vi "sv_UFF58 Create Function and Channels.vi"(0 "file refnum":refnum<k20>, 1 "real or complex data?":enum16{"Real data", "Complex data"}(ring), 11 "error in (no error)":errorcluster) -> (4 "dup file refnum":refnum<k20>, 6 "function refnum":refnum<k20>, 8 "channel refnums":refnum<k20>[](array[refnum]), 12 "ordinate denominator channel name":string, 13 "ordinate numerator channel name":string, 14 "abscissa channel name":string, 15 "error out":errorcluster)   [LabVIEW 2017, in "SoundVib_UFF58.lvlib"]
doc: "This VI creates a new <B>function refnum</B>. It also creates multiple <B>channel refnums</B> depending on the value of <B>real or complex data?</B>. If real, only two channels are created (X and Y). If complex, three channels are created (X, Yreal, and Yimag)."
uses:
  <vilib>/addons/Sound and Vibration/svt_UFF58/SoundVib_UFF58.lvlib
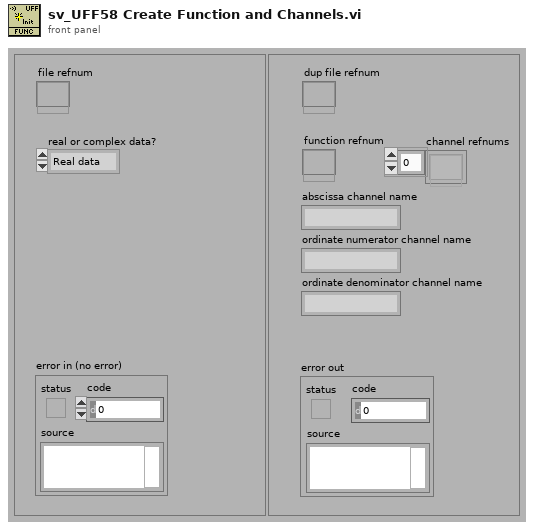
[diagram p1: front panel]
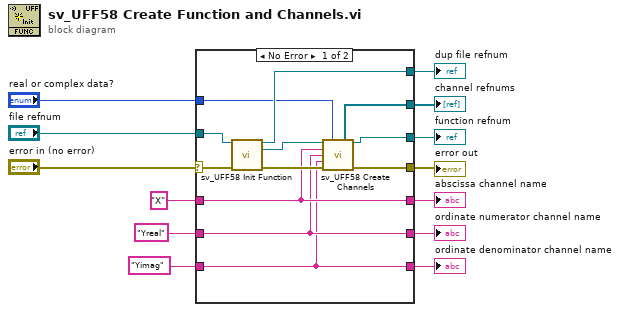
[diagram p0: block diagram]
diagram:
  n1 = case shown="No Error" "error in (no error)" {
    selector: "error in (no error)" -> [w19 w29]
    tunnel: "file refnum" -> [w25 w30]
    tunnel: [w24 w30] -> w12
    tunnel: "real or complex data?" -> [w22 _]
    tunnel: [w21 _] -> w10
    tunnel: [w17 _] -> w9
    tunnel: [w20 w29] -> w8
    tunnel: [w16 w28] -> w6
    tunnel: "X" ("abscissa channel name in") -> [w16 w28]
    tunnel: "Yreal" ("ordinate numerator channel name in") -> [w15 w27]
    tunnel: "Yimag" ("ordinate denominator channel name in") -> [w14 w26]
    tunnel: [w15 w27] -> w2
    tunnel: [w14 w26] -> w1
    frame No Error {
      n2 = call <vilib>:"sv_UFF58 Init Function.vi"("file refnum"=w25, "error in (no error)"=w19) -> ("dup file refnum"=w24:refnum<k20>, "function refnum"=w18:refnum<k20>, "error out"=w23:errorcluster)  [unwired: 11 in]
      n3 = call <vilib>:"sv_UFF58 Create Channels.vi"("function refnum"=w18, "real or complex data?"=w22, "abscissa channel name in"=w16, "ordinate numerator channel name in"=w15, "ordinate denominator channel name in"=w14, "error in (no error)"=w23) -> ("channel refnums"=w17:refnum<k20>[], "dup function refnum"=w21:refnum<k20>, "error out"=w20:errorcluster)  [unwired: 4 in, 3 out]
    }
    frame Error {
    }
  }
  "dup file refnum" <- w12
  "function refnum" <- w10
  "channel refnums" <- w9
  "error out" <- w8
  "abscissa channel name" <- w6
  "ordinate numerator channel name" <- w2
  "ordinate denominator channel name" <- w1
